vi "ReadArrayKeyence.vi"(8 "numDatos":i32=1 min=1, 9 "numero":i32, 10 "DataType Int":T1, 11 "connection ID":refnum<k5>) -> (0 "error out":errorcluster, 1 "datoB":string, 2 "datoA":string, 3 "connection ID out":refnum<k5>, 4 "length":i32)   [LabVIEW 2016]
uses:
  controlIntDataType.ctl
panel:
  out "concatenated string":string
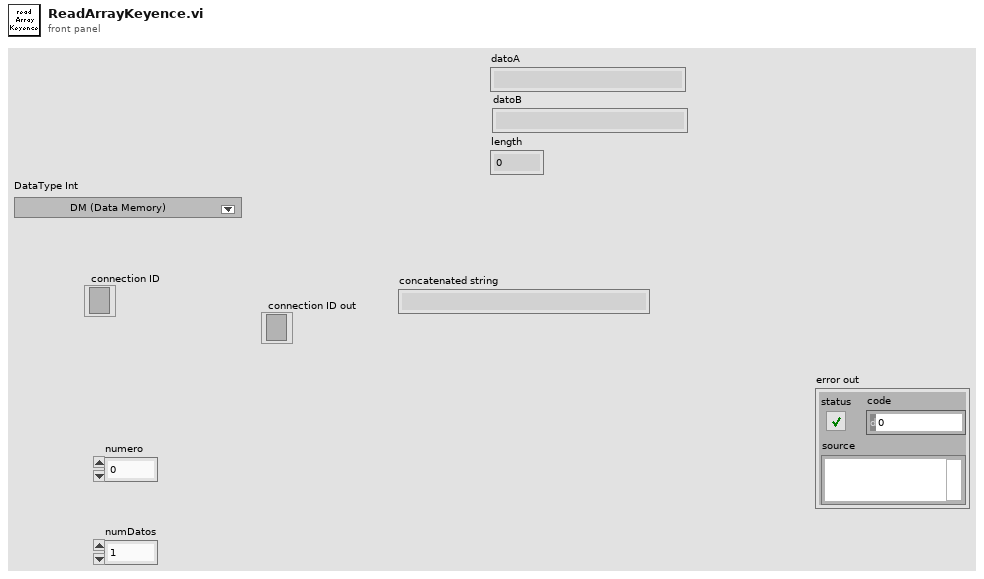
[diagram p1: front panel]
types:
  T1 = typedef "controlIntDataType.ctl" = u16
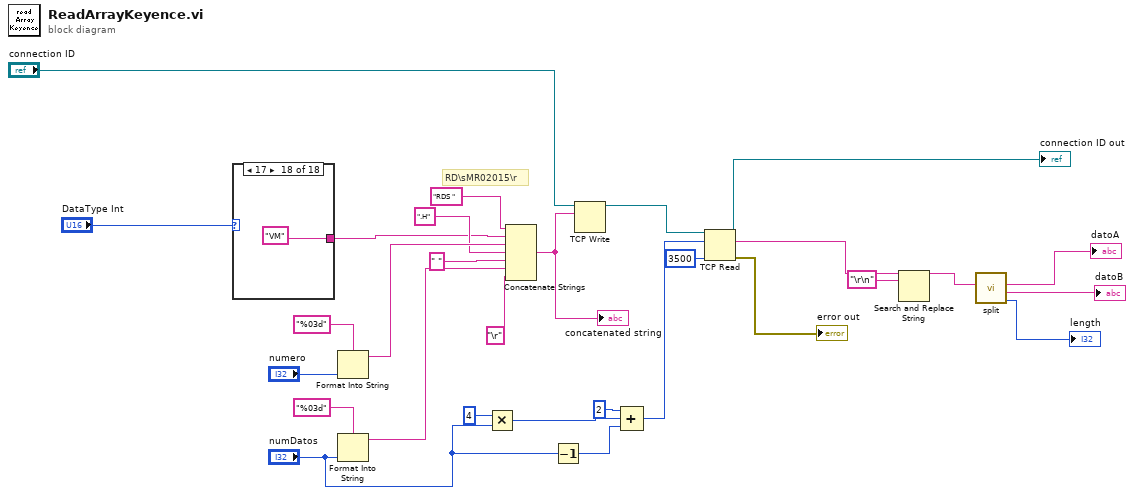
[diagram p0: block diagram]
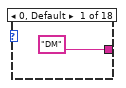
[diagram p2: hidden frame]
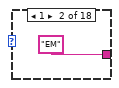
[diagram p3: hidden frame]
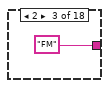
[diagram p4: hidden frame]
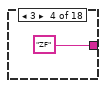
[diagram p5: hidden frame]
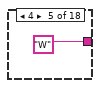
[diagram p6: hidden frame]
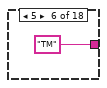
[diagram p7: hidden frame]
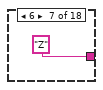
[diagram p8: hidden frame]
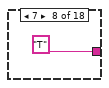
[diagram p9: hidden frame]
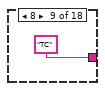
[diagram p10: hidden frame]
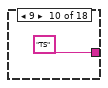
[diagram p11: hidden frame]
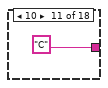
[diagram p12: hidden frame]
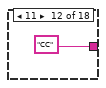
[diagram p13: hidden frame]
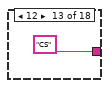
[diagram p14: hidden frame]
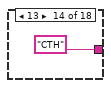
[diagram p15: hidden frame]
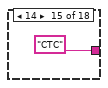
[diagram p16: hidden frame]
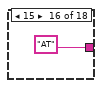
[diagram p17: hidden frame]
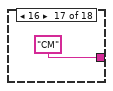
[diagram p18: hidden frame]
diagram:
  # "RD\\sMR02015\\r"
  n1 = case shown="17" "DataType Int" {
    tunnel: ["DM" ("string") "EM" ("string") "FM" ("string") "ZF" ("string") "W" ("string") "TM" ("string") "Z" ("string") "T" ("string") "TC" ("string") "TS" ("string") "C" ("string") "CC" ("string") "CS" ("string") "CTH" ("string") "CTC" ("string") "AT" ("string") "CM" ("string") "VM" ("string")] -> w18
    frame 0, Default {
    }
    frame 1 {
    }
    frame 2 {
    }
    frame 3 {
    }
    frame 4 {
    }
    frame 5 {
    }
    frame 6 {
    }
    frame 7 {
    }
    frame 8 {
    }
    frame 9 {
    }
    frame 10 {
    }
    frame 11 {
    }
    frame 12 {
    }
    frame 13 {
    }
    frame 14 {
    }
    frame 15 {
    }
    frame 16 {
    }
    frame 17 {
    }
  }
  n2 = Format Into String(format string="%03d", "numero") -> (resulting string=w21:string)  [unwired: 2 in, 1 out]
  n3 = Format Into String(format string="%03d", "numDatos") -> (resulting string=w14:string)  [unwired: 2 in, 1 out]
  n4 = Multiply(x=4, y="numDatos") -> (x*y=w11:i32)
  n5 = Concatenate Strings("RDS " ("string"), w18, w21, ".H" ("string"), " " ("string"), w14, "\r" ("string")) -> (w19:string)
  "concatenated string" <- w19
  n6 = Decrement(x="numDatos") -> (x-1=w7:i32)
  n7 = TCP Write(connection ID="connection ID", data in=w19) -> (connection ID out=w28:refnum<k5>)  [unwired: 2 in, 2 out]
  n8 = Compound Arithmetic op=ADD(2 ("x"), w11, w7) -> (w9:i32)
  n9 = TCP Read(connection ID=w28, bytes to read=w9, 9:3500 ("timeout ms (25000)")) -> (connection ID out=→"connection ID out":refnum<k5>, data out=w5:string, error out=→"error out":errorcluster)  [unwired: 2 in]
  n10 = Search and Replace String(input string=w5, search string="\r\n" ("format string")) -> (result string=w4:string)  [unwired: 6 in, 3 out]
  n11 = call "split.vi"("strInput"=w4) -> ("length"=→"length":i32, "datoB"=→"datoB":string, "datoA"=→"datoA":string)  [unwired: 8 in]
